vi "validate line configuration.vi"(7 "CVT configuration":refnum<class "CVT configuration.lvclass">, 11 "line in":T1) -> (1 "error":string, 2 "valid?":bool, 3 "line out":T1)   [LabVIEW 2013, in "CVT editor node.lvclass"]
uses:
  CVT editor node.lvclass
  table line.ctl
  <vilib>/NI/Tag Bus Module Framework/channel/TBM channel.lvclass
  configuration/CVT configuration.lvclass
  <vilib>/NI/Tag Bus/tag/tag descriptor.lvclass/tag descriptor.ctl
  <vilib>/NI/Tag Bus/tag/read tag name.vi
  <vilib>/NI/Tag Bus/tag/tag descriptor.lvclass
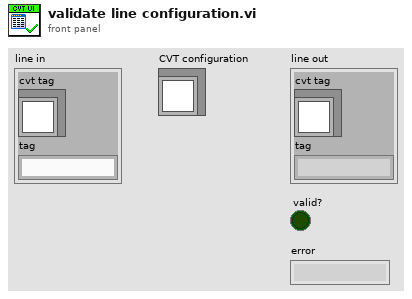
[diagram p1: front panel]
types:
  T1 = typedef "CVT editor node.lvclass/table line.ctl" = cluster{"cvt tag":refnum<class "TBM channel.lvclass">, "tag":string}
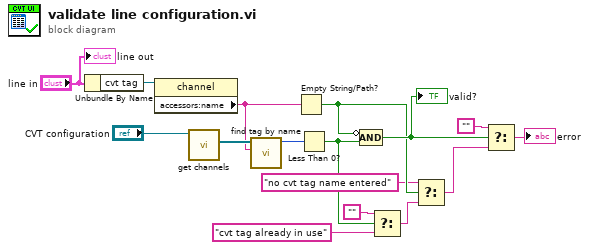
[diagram p0: block diagram]
diagram:
  n1 = Unbundle By Name("line in") -> ("cvt tag"=w15:refnum<class "TBM channel.lvclass">)
  n2 = property class="channel"(reference=w15) -> ("accessors:name"=w12:string)  [unwired: 1 in, 2 out]
  n3 = call-dynamic "get channels.vi"("CVT configuration in"="CVT configuration") -> ("channels"=w13:refnum<class "TBM channel.lvclass">[])  [unwired: 9 in, 1 out]
  n4 = call <vilib>:"find tag by name.vi"("name"=w12, "tags in"=w13) -> ("index"=w11:i32)  [unwired: 9 in]
  n5 = Empty String/Path?(string/path=w12) -> (empty?=w7:bool)
  n6 = Less Than 0?(x=w11) -> (x < 0?=w4:bool)
  n7 = Compound Arithmetic op=AND(invert w7, w4) -> (w10:bool)
  "valid?" <- w10
  n8 = Select(t="", s=w4, f="cvt tag already in use") -> (s? t:f=w1:string)
  n9 = Select(t="no cvt tag name entered", s=w7, f=w1) -> (s? t:f=w5:string)
  n10 = Select(t="", s=w10, f=w5) -> (s? t:f=→"error":string)
  "line out" <- "line in"
